vi "Validate Configuration Metadata.vi"(8 "error in (no error)":errorcluster, 11 "Measurement":refnum<class "MeasurementPluginService.lvclass">) -> (0 "error out":errorcluster, 2 "Invalid Parameters":string, 3 "Is Metadata Valid":bool)   [LabVIEW 2020, in "MeasurementLink Measurement Server.lvlib"]
uses:
  MeasurementLink Measurement Server.lvlib
  <vilib>/Utility/Data Type/NI_Data Type.lvlib
  Classes/MeasurementPluginService/MeasurementPluginService.lvclass
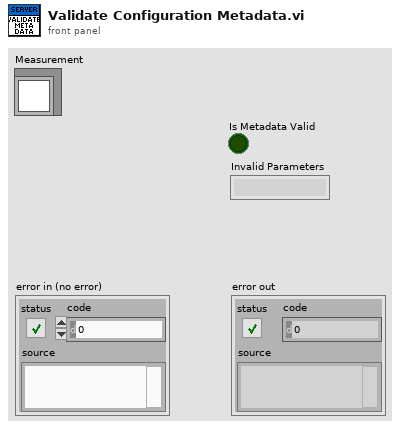
[diagram p1: front panel]
types:
  T1 = typedef "MeasurementLink Measurement Server.lvlib/MeasurementPluginService.lvclass/Plugin Paths.ctl" = cluster{"Get Measurement Details VI Path":path, "Get Type Specializations VI Path":path, "Measurement Logic VI Path":path, "Measurement Configuration CTL Path":path, "Measurement Results CTL Path":path, "Measurement UI VI Path":path}
  T2 = typedef "MeasurementLink Measurement Server.lvlib/Parameter Type Specialization.ctl" = cluster{"Parameter Name":string, "Type Specialization":T3, "Annotations":cluster{"Key":T4, "Value":string}[]}
  T3 = typedef "MeasurementLink Measurement Server.lvlib/Type Specialization.ctl" = enum16{"none", "pin"}
  T4 = typedef "MeasurementLink Measurement Server.lvlib/Key.ctl" = enum16{"none", "pin.instrument_type"}
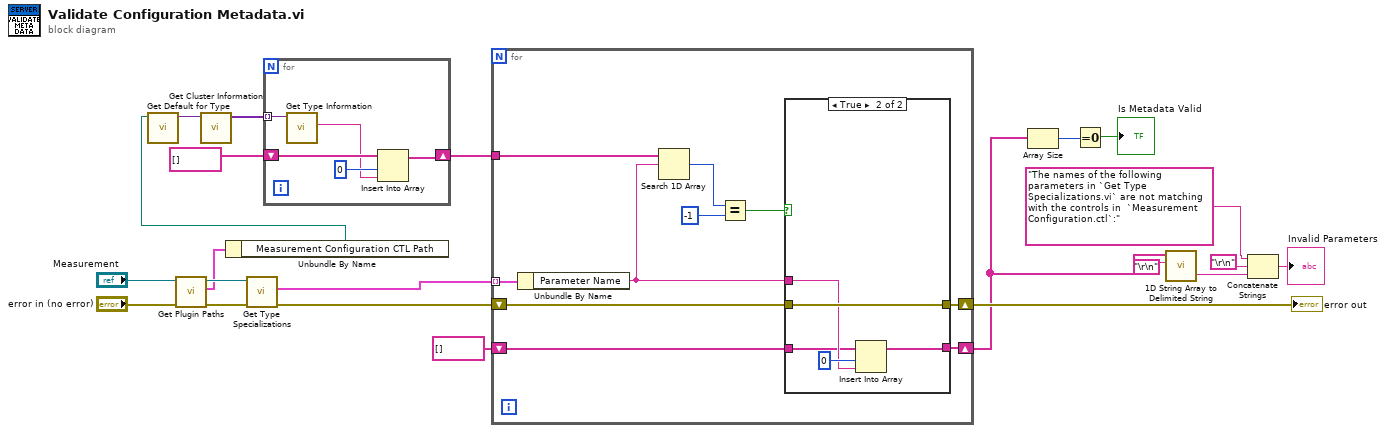
[diagram p0: block diagram]
diagram:
  n1 = call-dynamic "Get Plugin Paths.vi"("error in (no error)"="error in (no error)", "MeasurementService in"="Measurement") -> ("error out"=w5:errorcluster, "Plugin Paths"=w2:T1, "MeasurementService out"=w3:refnum<class "MeasurementPluginService.lvclass">)  [unwired: 7 in]
  n2 = Unbundle By Name(w2) -> ("Measurement Configuration CTL Path"=w1:path)
  n3 = call "Get Default for Type.vi"("Path of Type"=w1) -> ("Default for Type"=w9:variant)  [unwired: 9 in, 1 out]
  n4 = call <vilib>:"Get Cluster Information.vi"("variant"=w9) -> ("cluster elements"=w22:variant[])  [unwired: 9 in, 1 out]
  n5 = call-dynamic "Get Type Specializations.vi"("error in (no error)"=w5, "MeasurementService in"=w3) -> ("error out"=w8:errorcluster, "Type Specializations"=w7:T2[])  [unwired: 7 in, 1 out]
  n6 = for {
    tunnel: w22 -> [w27] mode=indexing
    shift-right: [w23] -> w20
    shift-left: string[] [] -> [w25]
    n7 = call <vilib>:"Get Type Information.vi"("variant"=w27) -> ("name"=w24:string)  [unwired: 6 in, 4 out]
    n8 = Insert Into Array(array=w25, index=0, new element=w24) -> (w23:string[])
  }
  n9 = for {
    tunnel: w7 -> [w37] mode=indexing
    shift-right: [w31] -> w18
    shift-left: w8 -> [w32]
    tunnel: w20 -> [w36]
    shift-right: [w28] -> w11
    shift-left: string[] [] -> [w30]
    n10 = Unbundle By Name(w37) -> ("Parameter Name"=w29:string)
    n11 = Search 1D Array(1D array=w36, element=w29) -> (index of element=w35:i32)  [unwired: 1 in]
    n12 = Equal?(x=w35, y=-1) -> (x = y?=w33:bool)
    n13 = case shown="True" w33 {
      tunnel: w32 -> [w39 w44]
      tunnel: [w39 w44] -> w31
      tunnel: w30 -> [w38 w41]
      tunnel: w29 -> [_ w42]
      tunnel: [w38 w40] -> w28
      frame False {
      }
      frame True {
        n14 = Insert Into Array(array=w41, index=0, new element=w42) -> (w40:string[])
      }
    }
  }
  "error out" <- w18
  n15 = Array Size(array=w11) -> (size(s)=w17:i32)
  n16 = Equal To 0?(x=w17) -> (x = 0?=→"Is Metadata Valid":bool)
  n17 = call <vilib>:"1D String Array to Delimited String.vi"("delimiter"="\r\n", "string array"=w11) -> ("delimited string"=w12:string)  [unwired: 9 in]
  n18 = Concatenate Strings("The names of the following parameters in `Get Type Specializations.vi` are not matching with the controls in  `Measurement Configuration.ctl`:" ("string"), "\r\n", w12) -> (→"Invalid Parameters":string)
